vi "create.vi"(8 "error in (no error)":errorcluster, 11 "MessageInterface in":refnum<class "MessageInterface.lvclass">) -> (0 "error out":errorcluster, 3 "MessageInterface out":refnum<class "MessageInterface.lvclass">, 10 "Parameters":variant)   [LabVIEW 2022 SP3, in "MessageInterface.lvclass"]
uses:
  MessageInterface.lvclass
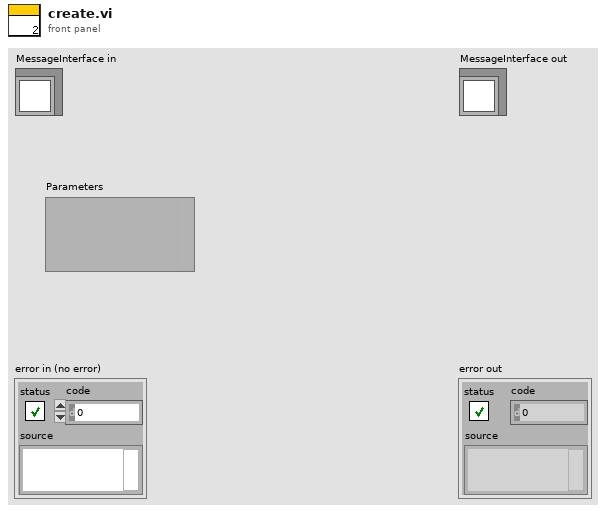
[diagram p1: front panel]
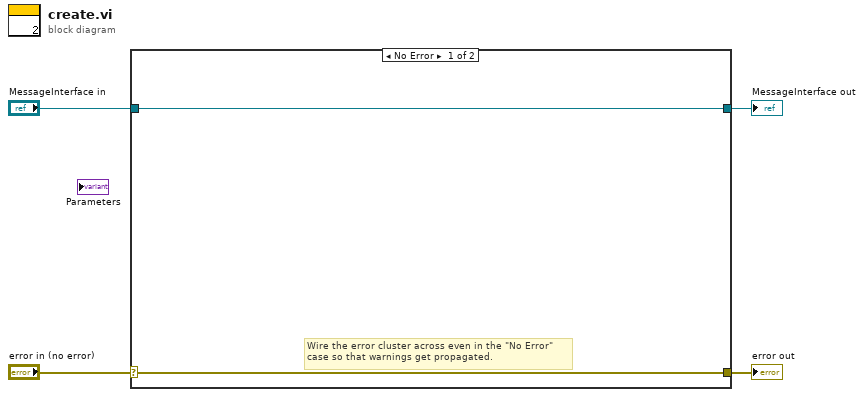
[diagram p0: block diagram]
diagram:
  n1 = case shown="No Error" "error in (no error)" {
    selector: "error in (no error)" -> [w5 w8]
    tunnel: [w5 w8] -> w3
    tunnel: [w6 w7] -> w1
    tunnel: "MessageInterface in" -> [w6 w7]
    frame No Error {
      # "Wire the error cluster across even in the \"No Error\"\ncase so that warnings get propagated."
    }
    frame Error {
    }
  }
  "error out" <- w3
  "MessageInterface out" <- w1
